vi "I2C Grove 64x48OLED_SSD1306_Graph.vi"() -> ()   [LabVIEW 2020, in "CTI-Scratchpad.lvlib"]
uses:
  CTI-Scratchpad.lvlib
  CTI/Identity.ctl
  CTI/Error Reporting.ctl
  CTI/GPIO Number.ctl
  CTI/I2C Number.ctl
  <vilib>/picture/cartesn2.llb/XY Plot Type.ctl
  CTI/Session/Session.lvclass
  CTI-Peripheral/I2C OLED/48x64 I2C OLED SSD1306/48x64 I2C OLED SSD1306.lvclass
  CTI/VisaComms/VisaComms.lvclass
  CTI/CTI.lvlib
panel:
  out "Identity":T1
  in  "stop":bool
  in  "Grove Connector":enum16{"I2C0", "I2C1"}(ring)
  out "2D Picture":picture
  out "error out":errorcluster
  in  "Port":refnum<visa-resource-name>="COM4"
  # "https://wiki.seeedstudio.com/Grove-OLED-Display-0.66-SSD1306_v1.0/"
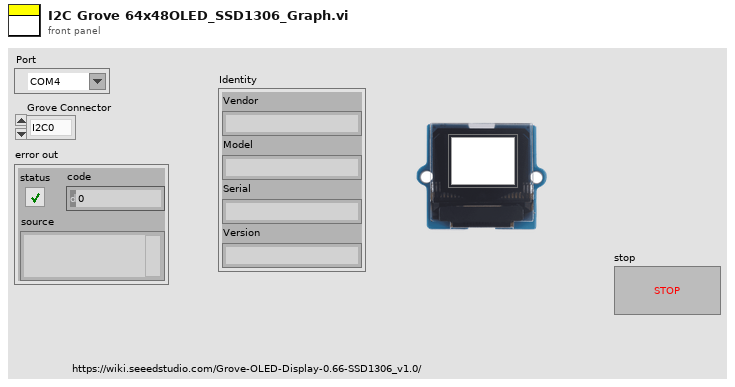
[diagram p1: front panel]
types:
  T1 = typedef "CTI.lvlib/Identity.ctl" = cluster{"Vendor":string, "Model":string, "Serial":string, "Version":string}
  T2 = typedef "CTI.lvlib/Error Reporting.ctl" = enum16{"Minimal", "Moderate", "Full"}
  T3 = typedef "CTI.lvlib/I2C Number.ctl" = i8
  T4 = typedef "CTI.lvlib/GPIO Number.ctl" = i8
  T5 = cluster{"Font Name:":string, "Size":i16, "Strikeout?":bool, "Italic?":bool, "Underline?":bool, "Outline?":bool, "Shadow?":bool, "Bold?":bool}
  T6 = cluster{"line color":u32, "text color":u32, "tick length(3)":i16, "crossing axes":bool, "visible grid?":bool}
  T7 = typedef "XY Plot Type.ctl" = enum16{"points", "squares", "circles", "connected points", "connected squares", "connected circles", "comb plot", "sized scatter plot", "sized-colored scatter plot", "min-max lines"}
  T8 = cluster{"plot color":u32, "XY plot type":T7, "baseline":dbl}
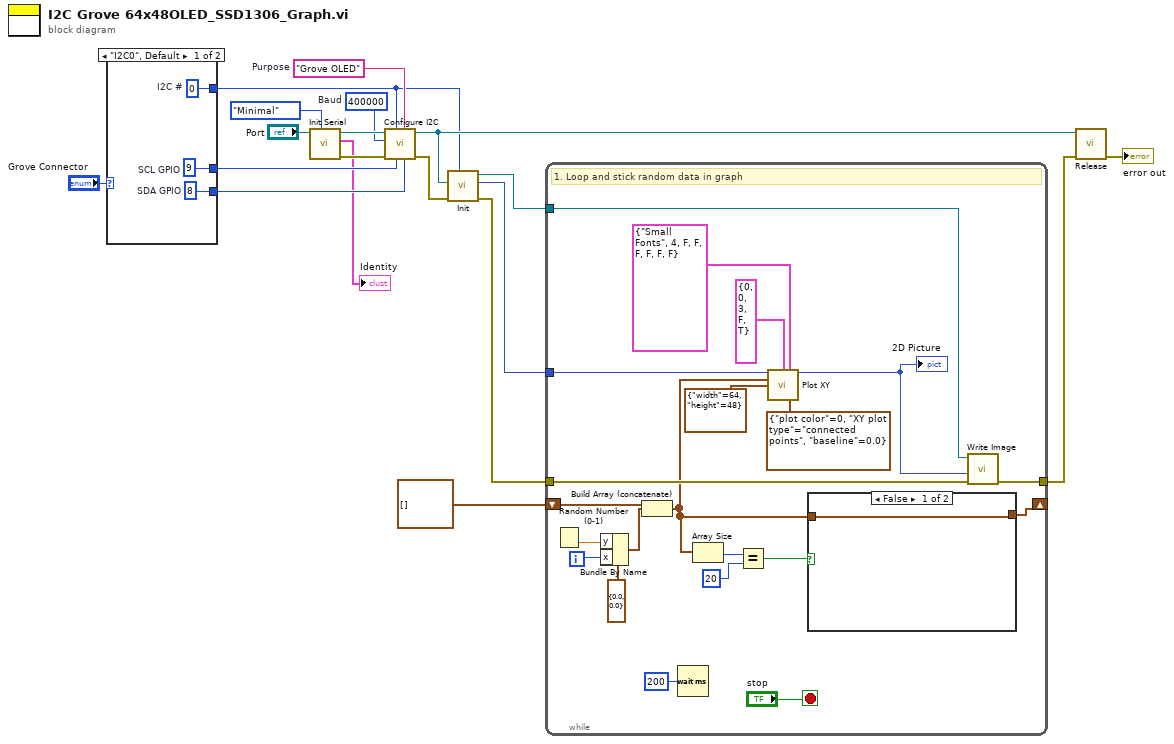
[diagram p0: block diagram]
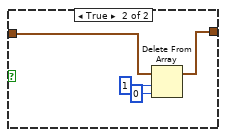
[diagram p2: hidden frame]
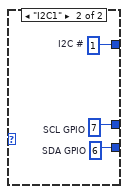
[diagram p3: hidden frame]
diagram:
  w14 = "Grove OLED"  # Purpose
  w15 = u32 400000  # Baud
  n1 = case shown="\"I2C0\", Default" "Grove Connector" {
    tunnel: [w22 w25] -> w10
    tunnel: [w21 w24] -> w9
    tunnel: [w20 w23] -> w8
    frame "I2C0", Default {
      w20 = T3 0  # I2C #
      w21 = T4 8  # SDA GPIO
      w22 = T4 9  # SCL GPIO
    }
    frame "I2C1" {
      w23 = T3 1  # I2C #
      w24 = T4 6  # SDA GPIO
      w25 = T4 7  # SCL GPIO
    }
  }
  n2 = call "Init Serial.vi"("Error Checking (Full)"=Error_Reporting."Minimal", "VISA resource name in"="Port") -> ("error out"=w16:errorcluster, "Identity"=→"Identity":T1, "Session"=w17:refnum<class "Session.lvclass">)  [unwired: 7 in]
  n3 = call "Configure I2C.vi"("SDA GPIO"=w9, "Purpose (\"I2C\")"=w14, "SCL GPIO"=w10, "I2C #"=w8, "error in (no error)"=w16, "Baud"=w15, "Session in"=w17) -> ("error out"=w13:errorcluster, "Session out"=w12:refnum<class "Session.lvclass">)  [unwired: 3 in]
  n4 = call "Init.vi"("I2C #"=w8, "error in (no error)"=w13, "Session In"=w12) -> ("error out"=w3:errorcluster, "2D Picture"=w5:picture, "48x64 I2C OLED SSD1306 Out"=w4:refnum<class "48x64 I2C OLED SSD1306.lvclass">)  [unwired: 6 in]
  n5 = while {
    tunnel: w5 -> [w46]
    tunnel: w3 -> [w36]
    shift-right: [w26] -> _
    shift-left: cluster{"x":dbl, "y":dbl}[] [] ("data") -> [w41]
    tunnel: w4 -> [w37]
    tunnel: [w35] -> w2
    i -> [w43]
    stop <- "stop" stop-if-true
    # "1. Loop and stick random data in graph"
    n6 = Random Number (0-1)() -> (number: 0 to 1=w42:dbl)
    n7 = Bundle By Name(cluster=cluster{"x":dbl, "y":dbl} {"x"=0.0, "y"=0.0} ("Point [horizontal, vertical]"), "y"=w42, "x"=w43) -> (w40:cluster{"x":dbl, "y":dbl})
    n8 = Build Array (concatenate)(w41, w40) -> (w27:cluster{"x":dbl, "y":dbl}[])
    n9 = Wait (ms)(milliseconds to wait=u32 200) -> ()  [unwired: 1 out]
    n10 = Array Size(array=w27) -> (size(s)=w30:i32)
    n11 = Equal?(x=w30, y=20) -> (x = y?=w28:bool)
    n12 = call <vilib>:"Plot XY.vi"("picture"=w46, "[user-specified font]"=T5 {"Font Name:"="Small Fonts", "Size"=4, "Strikeout?"=FALSE, "Italic?"=FALSE, "Underline?"=FALSE, "Outline?"=FALSE, "Shadow?"=FALSE, "Bold?"=FALSE}, "data"=w27, "dimensions (w,h)"=cluster{"width":i16, "height":i16} {"width"=64, "height"=48}, "cartesian grid cosmetics"=T6 {"line color"=0, "text color"=0, "tick length(3)"=3, "crossing axes"=FALSE, "visible grid?"=TRUE}, "XY plot cosmetics"=T8 {"plot color"=0, "XY plot type"=enum."connected points", "baseline"=0.0}) -> ("new picture"=w32:picture)  [unwired: 9 in]
    "2D Picture" <- w32
    n13 = case shown="False" w28 {
      tunnel: w27 -> [w47 w51]
      tunnel: [w47 w50] -> w26
      frame False {
      }
      frame True {
        n14 = Delete From Array(array=w51, length=1, index=0) -> (array with subset deleted=w50:cluster{"x":dbl, "y":dbl}[])  [unwired: 1 out]
      }
    }
    n15 = call-dynamic "Write Image.vi"("error in (no error)"=w36, "2D Picture"=w32, "48x64 I2C OLED SSD1306 In"=w37) -> ("error out"=w35:errorcluster)  [unwired: 7 in, 1 out]
  }
  n16 = call-dynamic "Release.vi"("error in (no error)"=w2, "Session in"=w12) -> ("error out"=→"error out":errorcluster)  [unwired: 9 in]
